vi "Reset.vi"(8 "error in (no error)":errorcluster, 11 "Osciloscope in":refnum<class "Osciloscope.lvclass">) -> (0 "error out":errorcluster, 3 "Osciloscope out":refnum<class "Osciloscope.lvclass">)   [LabVIEW 2020, in "Controlador.lvlib" / "Osciloscope.lvclass"]
uses:
  Osciloscope.lvclass
  Osciloscope.lvclass/Osciloscope.ctl
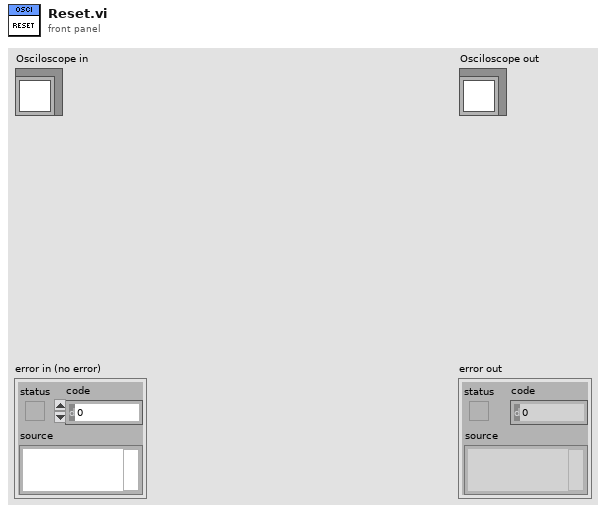
[diagram p1: front panel]
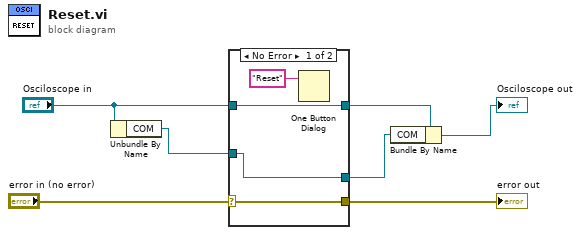
[diagram p0: block diagram]
diagram:
  n1 = Unbundle By Name("Osciloscope in") -> ("COM"=w4:refnum<visa-resource-name>)
  n2 = case shown="No Error" "error in (no error)" {
    selector: "error in (no error)" -> [w10 w13]
    tunnel: [w10 w13] -> w6
    tunnel: [w11 w12] -> w3
    tunnel: "Osciloscope in" -> [w11 w12]
    tunnel: w4 -> [w9 _]
    tunnel: [w9 _] -> w1
    frame No Error {
      n3 = One Button Dialog(message="Reset") -> ()  [unwired: 1 in, 1 out]
    }
    frame Error {
    }
  }
  "error out" <- w6
  n4 = Bundle By Name(cluster=w3, "COM"=w1) -> (→"Osciloscope out":refnum<class "Osciloscope.lvclass">)
